vi "data_acqui.vi"() -> ()   [LabVIEW 2019]
uses:
  <vilib>/Utility/error.llb/DialogType.ctl
  <vilib>/DAQmx/write.llb/DAQmx Write (Counter Frequency 1Chan 1Samp).vi
  <vilib>/DAQmx/create/channels.llb/DAQmx Create Channel (CO-Pulse Generation-Frequency).vi
  <vilib>/DAQmx/configure/timing.llb/DAQmx Timing (Implicit).vi
  <vilib>/DAQmx/miscellaneous.llb/DAQmx Fill In Error Info.vi
  <vilib>/Utility/file.llb/Write Delimited Spreadsheet (string).vi
  <instrlib>/Agilent 34970/Agilent 34970.lvlib
  <resource>/objmgr/daqmx.rc
panel:
  out "Waveform Chart":cluster{dbl, dbl}(graph)
  in  "stop geral":bool
  in  "Liga aquecedor":bool
  in  "Frequency":dbl=1.0 format="%.6f"
  in  "Duty Cycle":sgl=0.1 min=0.1 max=99.9 format="%#_6f"
  in  "Identifier":string
  in  "STOP":bool
  out "Interation":i32
  out "Time":dbl=300.0 format="%<%H:%M:%S>t"
  out "Temperature CH9 [degC]":dbl
  out "Temperature CH4 [degC]":dbl
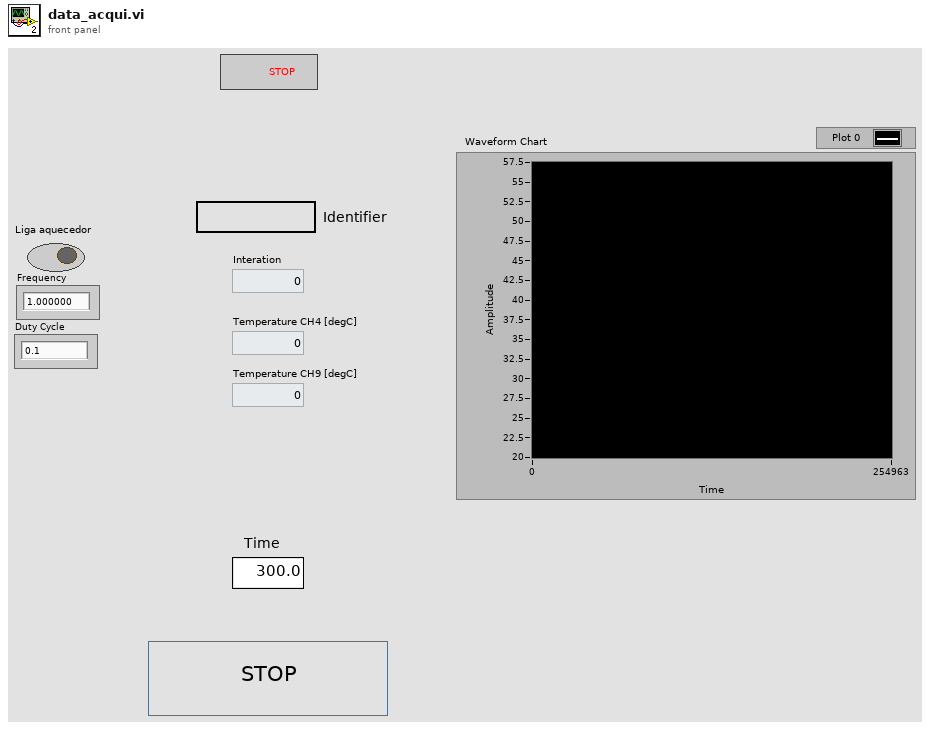
[diagram p1: front panel]
types:
  T1 = enum16{"Thermocouple", "Thermistor", "RTD", "4-Wire RTD", "Default (Last)"}
  T2 = typedef "DialogType.ctl" = u16
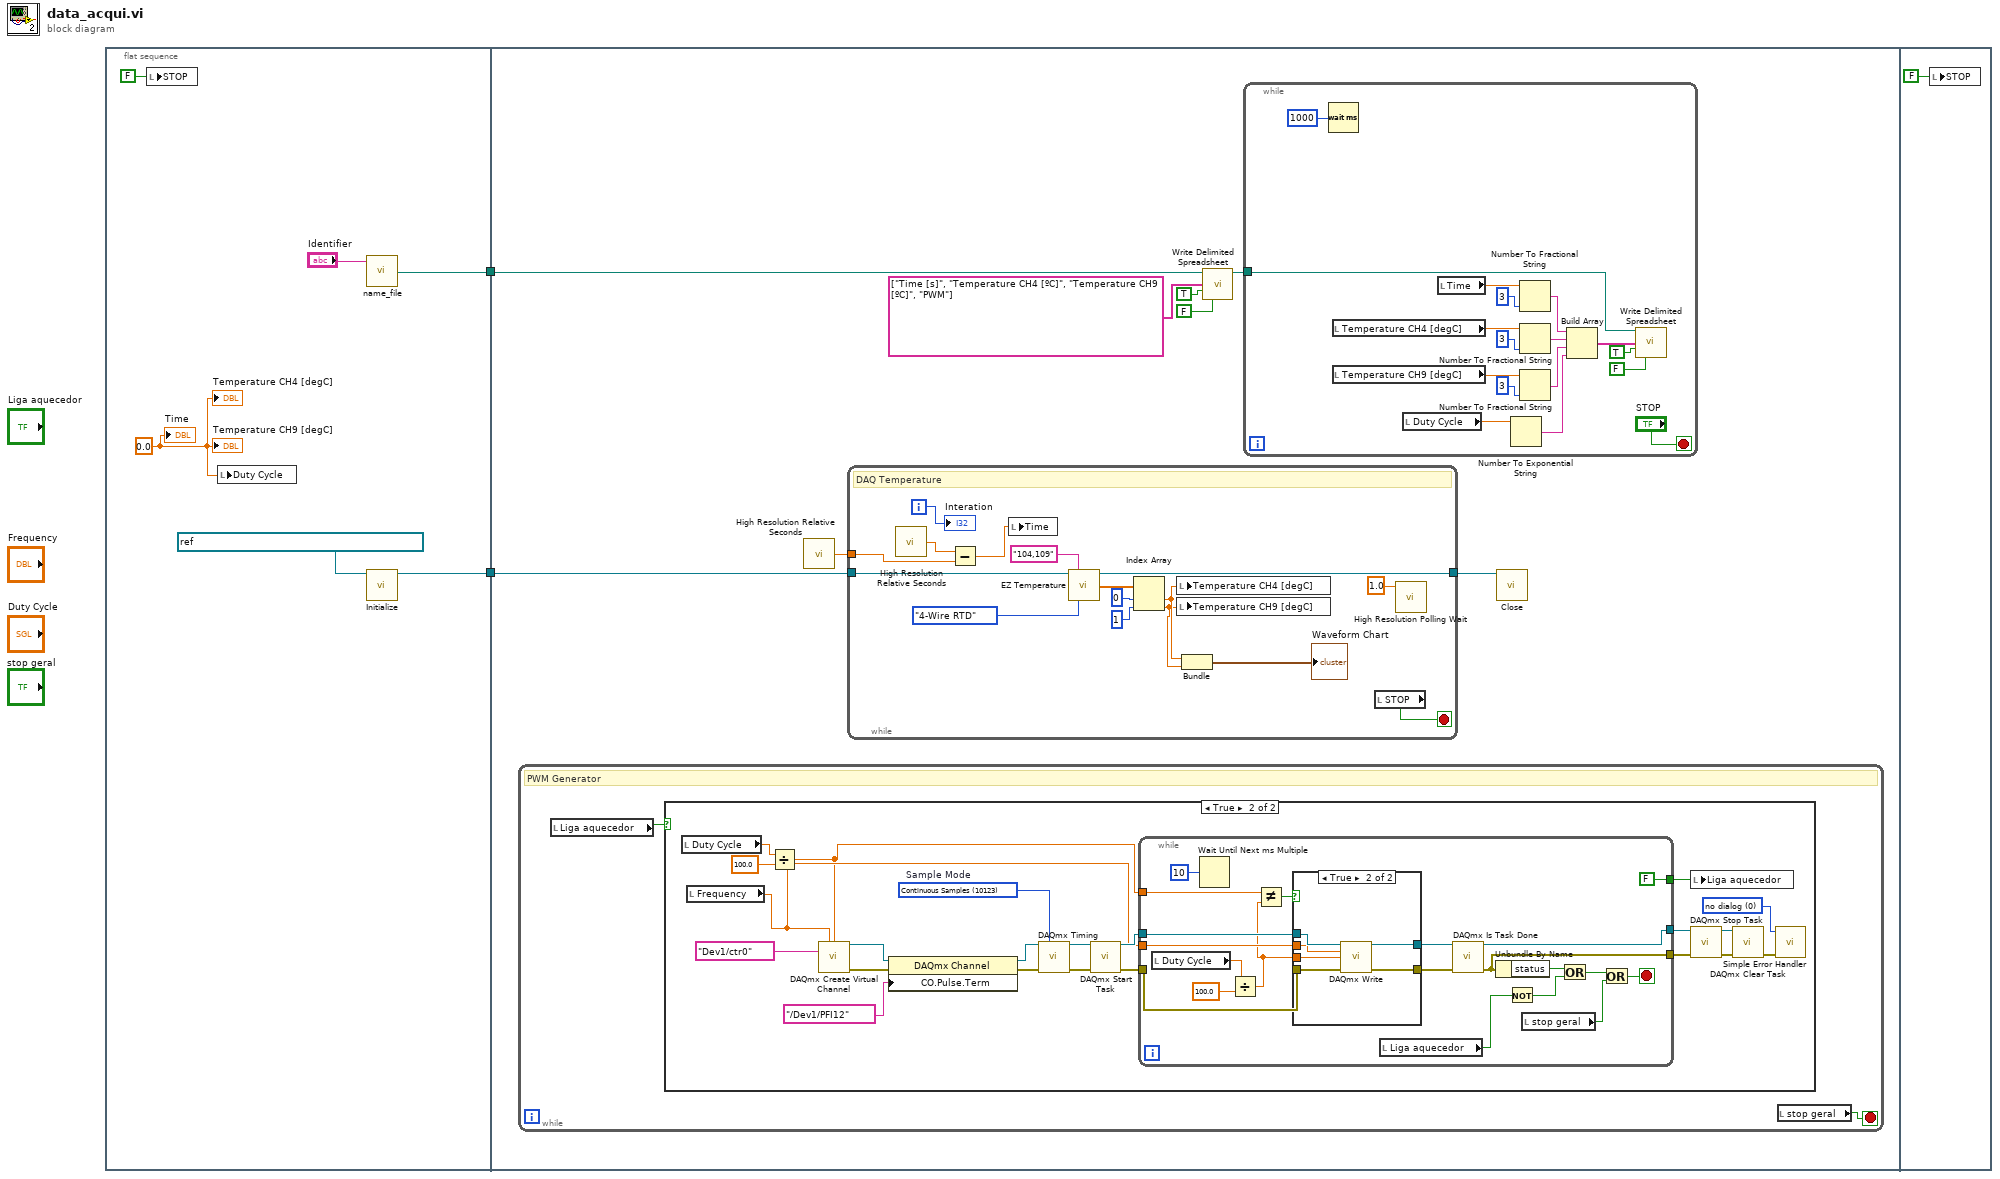
[diagram p0: block diagram]
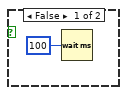
[diagram p2: hidden frame]
diagram:
  n1 = flat-sequence {
    tunnel: [w6] -> w2
    tunnel: [w5] -> w1
    tunnel: w2 -> [w14]
    tunnel: w1 -> [w9]
    frame #0 {
      w8 = 0.0 ("Temperature 1")
      n2 = local write "STOP"(FALSE ("STOP")) -> ()
      n3 = local write "Duty Cycle"(w8) -> ()
      n4 = call "name_file.vi"("Identifier"="Identifier") -> ("appended path"=w5:path)  [unwired: 2 in]
      n5 = call <instrlib>:"Initialize.vi"("VISA Resource Name"=refnum<visa-resource-name> "USB0::0x0957::0x2007::MY49006789::INSTR" ("VISA AGILENT")) -> ("VISA Resource Name Out"=w6:refnum<visa-resource-name>)  [unwired: 13 in, 1 out]
      "Temperature CH4 [degC]" <- w8
      "Temperature CH9 [degC]" <- w8
      "Time" <- w8
    }
    frame #1 {
      n6 = while {
        stop <- w17 stop-if-true
        # "PWM Generator"
        n7 = local read "Liga aquecedor"() -> (w18:bool)
        n8 = case shown="True" w18 {
          frame False {
            n9 = Wait (ms)(milliseconds to wait=u32 100) -> ()  [unwired: 1 out]
          }
          frame True {
            w26 = T2 0 items=["no dialog", "OK message", "continue or stop message", "OK message + warnings", "continue/stop + warnings"] ("type of dialog (OK msg:1)")
            w37 = 10123 items=["Finite Samples"=10178, "Continuous Samples"=10123, "Hardware Timed Single Point"=12522]  # Sample Mode
            n10 = local read "Duty Cycle"() -> (w21:sgl)
            n11 = local read "Frequency"() -> (w23:dbl)
            n12 = Divide(x=w21, y=100.0) -> (x/y=w20:dbl)
            n13 = call-poly <vilib>:"DAQmx Create Virtual Channel.vi"("frequency"=w23, "duty cycle"=w20, "counter"=tag "Dev1/ctr0" ("Counter")) -> ("task out"=w40:refnum<k21>, "error out"=w39:errorcluster)  [unwired: 11 in]
            n14 = property class="DAQmx Channel"(reference=w40, error in=w39, "CO.Pulse.Term"=tag "/Dev1/PFI12" ("Output Terminal")) -> (reference out=w36:refnum<k21>, error out=w35:errorcluster)
            n15 = call-poly <vilib>:"DAQmx Timing.vi"("task/channels in"=w36, "sample mode"=w37, "error in"=w35) -> ("task out"=w34:refnum<k21>, "error out"=w33:errorcluster)  [unwired: 11 in]
            n16 = call <vilib>:"DAQmx Start Task.vi"("task/channels in"=w34, "error in"=w33) -> ("task out"=w32:refnum<k21>, "error out"=w31:errorcluster)  [unwired: 12 in]
            n17 = while {
              tunnel: w32 -> [w51]
              tunnel: w31 -> [w49]
              tunnel: [w60] -> w28
              tunnel: [w61] -> w29
              tunnel: [FALSE ("Liga aquecedor")] -> w25
              tunnel: w20 -> [w47]
              tunnel: w23 -> [w45]
              stop <- w54 stop-if-true
              n18 = local read "Duty Cycle"() -> (w44:sgl)
              n19 = Wait Until Next ms Multiple(millisecond multiple=u32 10) -> ()  [unwired: 1 out]
              n20 = Divide(x=w44, y=100.0) -> (x/y=w42:dbl)
              n21 = Not Equal?(x=w47, y=w42) -> (x != y?=w46:bool)
              n22 = case shown="True" w46 {
                tunnel: [w63 w66] -> w50
                tunnel: w51 -> [w63 w67]
                tunnel: [w62 w68] -> w48
                tunnel: w49 -> [w62 w69]
                tunnel: w42 -> [_ w65]
                tunnel: w45 -> [_ w64]
                frame False {
                }
                frame True {
                  n23 = call-poly <vilib>:"DAQmx Write.vi"("task/channels in"=w67, "frequency"=w64, "duty cycle"=w65, "error in"=w69) -> ("task out"=w66:refnum<k21>, "error out"=w68:errorcluster)  [unwired: 9 in, 1 out]
                }
              }
              n24 = local read "Liga aquecedor"() -> (w57:bool)
              n25 = call <vilib>:"DAQmx Is Task Done.vi"("task/channels in"=w50, "error in"=w48) -> ("task out"=w61:refnum<k21>, "error out"=w60:errorcluster)  [unwired: 11 in, 1 out]
              n26 = Unbundle By Name(w60) -> ("status"=w59:bool)
              n27 = Not(x=w57) -> (.not. x?=w55:bool)
              n28 = local read "stop geral"() -> (w52:bool)
              n29 = Or(x=w59, y=w55) -> (x .or. y?=w53:bool)
              n30 = Or(x=w53, y=w52) -> (x .or. y?=w54:bool)
            }
            n31 = local write "Liga aquecedor"(w25) -> ()
            n32 = call <vilib>:"DAQmx Stop Task.vi"("task/channels in"=w29, "error in"=w28) -> ("task out"=w24:refnum<k21>, "error out"=w30:errorcluster)  [unwired: 12 in]
            n33 = call <vilib>:"DAQmx Clear Task.vi"("task in"=w24, "error in"=w30) -> ("error out"=w27:errorcluster)  [unwired: 13 in]
            n34 = call <vilib>:"Simple Error Handler.vi"("error code (no error:0)"=w26, "error in (no error)"=w27) -> ()  [unwired: 3 in, 5 out]
          }
        }
        n35 = local read "stop geral"() -> (w17:bool)
      }
      n36 = call <vilib>:"High Resolution Relative Seconds.vi"() -> ("relative seconds"=w16:dbl)
      n37 = while {
        tunnel: w14 -> [w98]
        tunnel: w16 -> [w99]
        tunnel: [w97] -> w15
        i -> [w101]
        stop <- w91 stop-if-true
        # "DAQ Temperature"
        n38 = call <vilib>:"High Resolution Relative Seconds.vi"() -> ("relative seconds"=w100:dbl)
        n39 = Subtract(x=w100, y=w99) -> (x-y=w92:dbl)
        n40 = local write "Time"(w92) -> ()
        n41 = call <instrlib>:"EZ Temperature.vi"("VISA Resource Name"=w98, "Scan List (empty)"="104,109", "Transducer Type (4:Def-Last)"=T1."4-Wire RTD") -> ("VISA Resource Name Out"=w97:refnum<visa-resource-name>, "Output Array"=w90:dbl[])  [unwired: 10 in, 1 out]
        n42 = Index Array(array=w90, index #1=0 ("index"), index #2=1 ("index")) -> (element #1=w89:dbl, element #2=w88:dbl)
        n43 = local write "Temperature CH4 [degC]"(w89) -> ()
        n44 = local write "Temperature CH9 [degC]"(w88) -> ()
        n45 = Bundle(w89, w88) -> (→"Waveform Chart":cluster{dbl, dbl})  [unwired: 1 in]
        n46 = local read "STOP"() -> (w91:bool)
        n47 = call <vilib>:"High Resolution Polling Wait.vi"("seconds to wait"=1.0) -> ()  [unwired: 10 in, 1 out]
        "Interation" <- w101
      }
      n48 = call-poly <vilib>:"Write Delimited Spreadsheet.vi"("file path (dialog if empty)"=w9, "1D data"=string[] ["Time [s]", "Temperature CH4 [ºC]", "Temperature CH9 [ºC]", "PWM"] ("appended array"), "append to file? (new file:F)"=TRUE, "transpose? (no:F)"=FALSE) -> ("new file path (Not A Path if cancelled)"=w10:path)  [unwired: 10 in, 1 out]
      n49 = while {
        tunnel: w10 -> [w84]
        stop <- "STOP" stop-if-true
        n50 = Wait (ms)(milliseconds to wait=u32 1000) -> ()  [unwired: 1 out]
        n51 = local read "Temperature CH4 [degC]"() -> (w79:dbl)
        n52 = local read "Temperature CH9 [degC]"() -> (w73:dbl)
        n53 = local read "Duty Cycle"() -> (w80:sgl)
        n54 = local read "Time"() -> (w77:dbl)
        n55 = Number To Exponential String(number=w80) -> (E-format string=w82:string)  [unwired: 3 in]
        n56 = Number To Fractional String(number=w77, precision (6)=i16 3) -> (F-format string=w76:string)  [unwired: 2 in]
        n57 = Number To Fractional String(number=w79, precision (6)=i16 3) -> (F-format string=w75:string)  [unwired: 2 in]
        n58 = Number To Fractional String(number=w73, precision (6)=i16 3) -> (F-format string=w71:string)  [unwired: 2 in]
        n59 = Build Array(w76, w75, w71, w82) -> (w72:string[])
        n60 = call-poly <vilib>:"Write Delimited Spreadsheet.vi"("file path (dialog if empty)"=w84, "1D data"=w72, "append to file? (new file:F)"=TRUE, "transpose? (no:F)"=FALSE) -> ()  [unwired: 10 in, 2 out]
      }
      n61 = call <instrlib>:"Close.vi"("VISA Resource Name"=w15) -> ()  [unwired: 14 in, 1 out]
    }
    frame #2 {
      n62 = local write "STOP"(FALSE ("STOP")) -> ()
    }
  }
